vi "DAQ Loop.vi"(8 "error in":errorcluster, 10 "Queues":T1, 11 "Notifiers":T2) -> (0 "error out":errorcluster)   [LabVIEW 2014, in "DAQ.lvlib"]
uses:
  DAQ.lvlib
  support/Message Queue/Message Queue.lvlib
  TypeDefs/DAQ data.ctl
  <vilib>/ErrorRing/Error Ring.xnode
  PLC/PLC.lvlib
  <vilib>/Utility/error.llb/Error Cluster From Error Code.vi
  Support/Global names.vi
  Support/Message Queue/Message Cluster.ctl
  Support/Notifiers/Notifiers.ctl
  Support/Notifiers/Notifiers.lvlib
  Support/Message Queue/All Message Queues.ctl
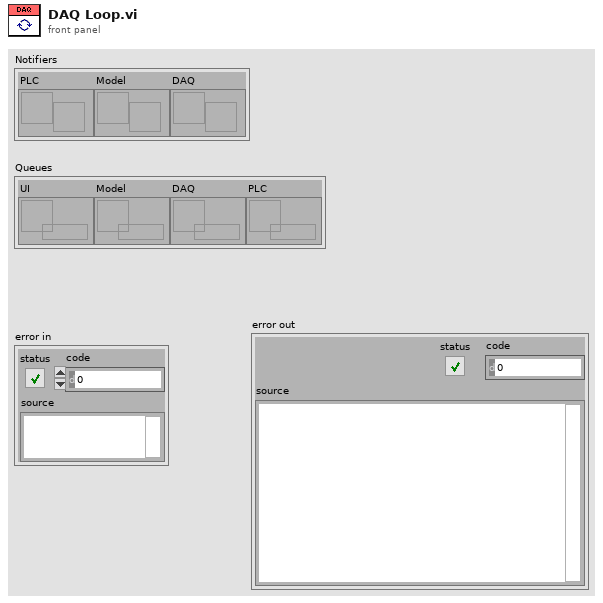
[diagram p1: front panel]
types:
  T1 = typedef "Message Queue.lvlib/All Message Queues.ctl" = cluster{"UI":refnum<queue>, "Model":refnum<queue>, "DAQ":refnum<queue>, "PLC":refnum<queue>}
  T2 = typedef "Notifiers.lvlib/Notifiers.ctl" = cluster{"PLC":refnum<notifier>, "Model":refnum<notifier>, "DAQ":refnum<notifier>}
  T3 = typedef "DAQ.lvlib/DAQ data.ctl" = cluster{"Power switch (DI)":cluster{"Channel":tag, "Data":bool}, "Dispose barrel (DI)":cluster{"Channel":tag, "Data":bool}, "Pump status (DO)":cluster{"Channel":tag, "Data":bool}, "Barrel position (AI)":cluster{"Channel":tag, "Data":dbl}}
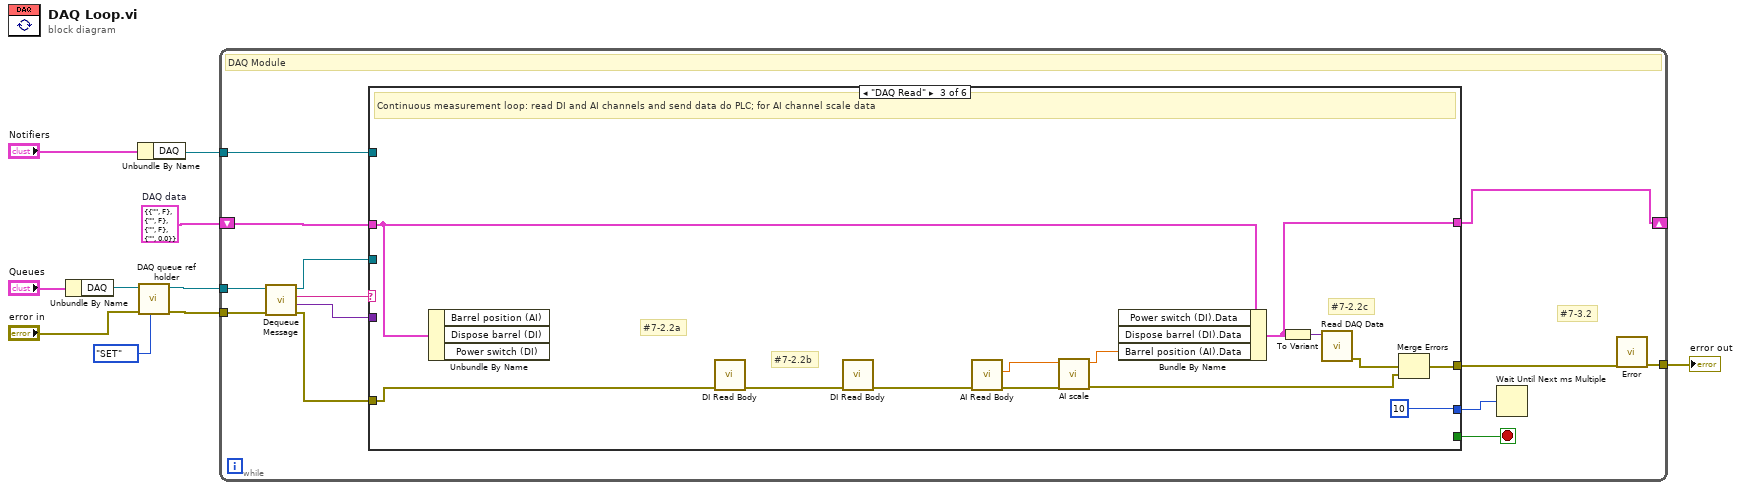
[diagram p0: block diagram]
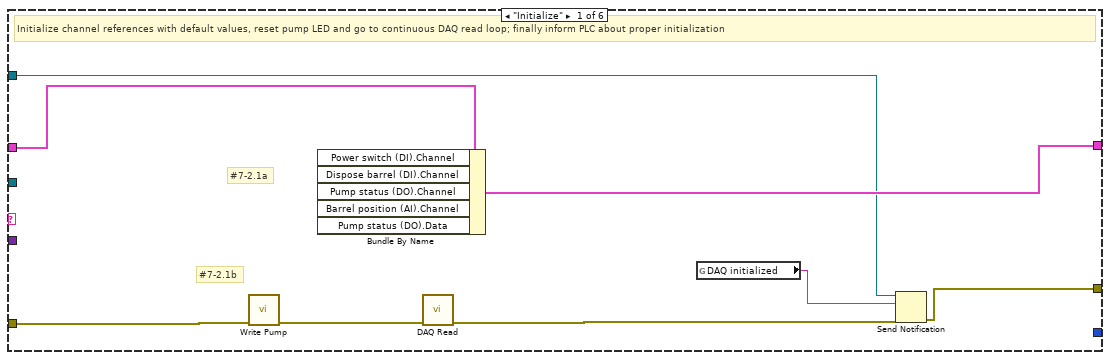
[diagram p2: hidden frame]
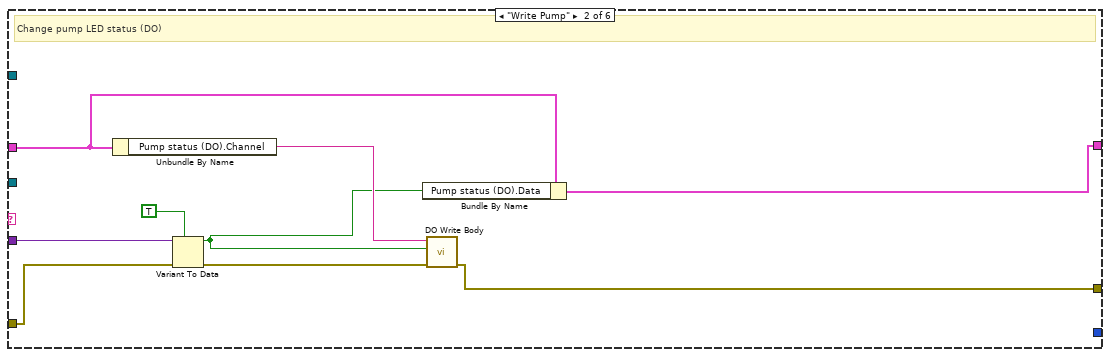
[diagram p3: hidden frame]
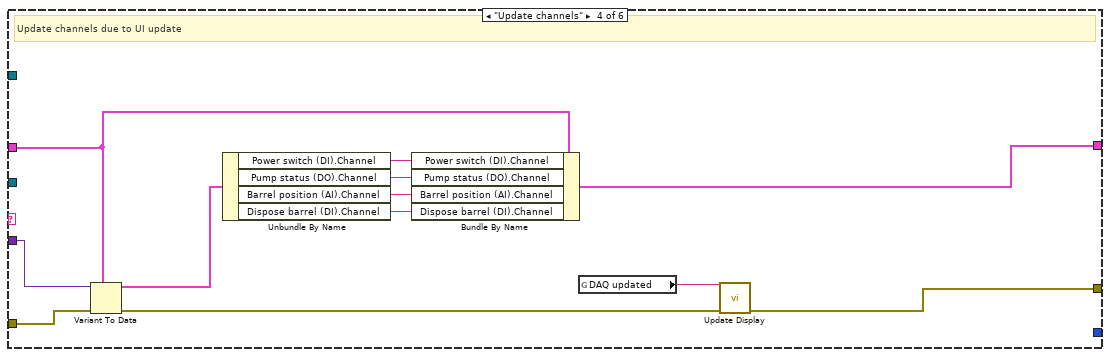
[diagram p4: hidden frame]
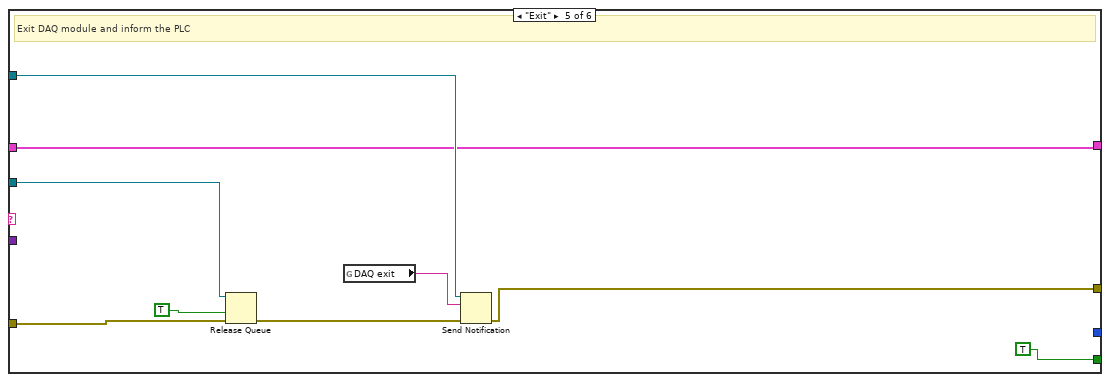
[diagram p5: hidden frame]
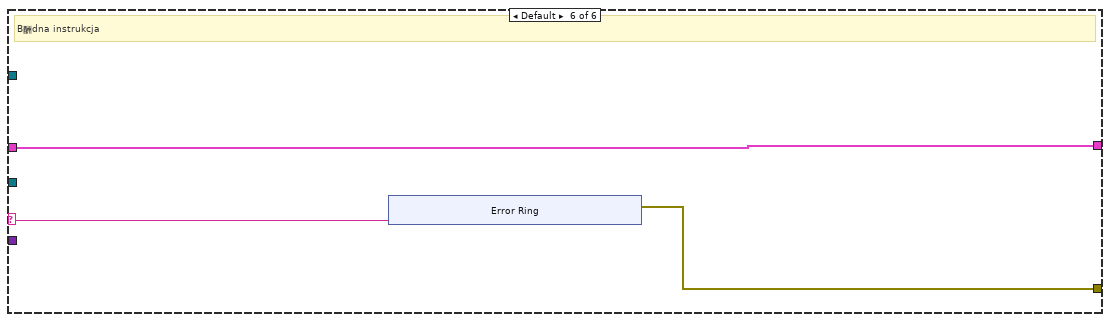
[diagram p6: hidden frame]
diagram:
  w10 = T3 {"Power switch (DI)"={"Channel"="", "Data"=FALSE}, "Dispose barrel (DI)"={"Channel"="", "Data"=FALSE}, "Pump status (DO)"={"Channel"="", "Data"=FALSE}, "Barrel position (AI)"={"Channel"="", "Data"=0.0}}  # DAQ data
  n1 = Unbundle By Name("Queues") -> ("DAQ"=w5:refnum<queue>)
  n2 = Unbundle By Name("Notifiers") -> ("DAQ"=w6:refnum<notifier>)
  n3 = call "DAQ queue ref holder.vi"("Action"=enum16{"GET", "SET"}."SET", "error in"="error in", "Message Queue In"=w5) -> ("error out"=w3:errorcluster, "Input Message Queue"=w4:refnum<queue>)  [unwired: 7 in]
  n4 = while {
    tunnel: w3 -> [w23]
    tunnel: w4 -> [w11]
    tunnel: w6 -> [w19]
    shift-right: [w18] -> _
    shift-left: w10 -> [w16]
    tunnel: [w14] -> w8
    stop <- w20 stop-if-true
    # "#7-3.2"
    # "DAQ Module"
    n5 = call "Dequeue Message.vi"("error in (no error)"=w23, "Message Queue"=w11) -> ("error out"=w22:errorcluster, "Message Data"=w21:variant, "Message"=w12:string, "dup Message Queue"=w13:refnum<queue>)  [unwired: 6 in]
    n6 = case shown="\"DAQ Read\"" w12 {
      selector: w12 -> [_ _ _ _ _ w76]
      tunnel: w22 -> [w28 w40 w46 w64 w68 _]
      tunnel: [w31 w32 w44 w56 w67 w75] -> w15
      tunnel: w21 -> [_ w39 _ w65 _ _]
      tunnel: [_ _ _ _ TRUE _] -> w20
      tunnel: w13 -> [_ _ _ _ w74 _]
      tunnel: w19 -> [w26 _ _ _ w73 _]
      tunnel: w16 -> [w30 w36 w51 w63 w69 w77]
      tunnel: [w29 w38 w48 w58 w69 w77] -> w18
      tunnel: [_ _ u32 10 ("millisecond multiple") _ _ _] -> w17
      frame "Initialize" {
        # "#7-2.1b"
        # "#7-2.1a"
        # "Initialize channel references with default values, reset pump LED and go to continuous DAQ read loop; finally inform PLC about proper initialization"
        n7 = call "Write Pump.vi"("error in"=w28) -> ("error out"=w27:errorcluster)  [unwired: 10 in]
        n8 = Bundle By Name(cluster=w30) -> (w29:T3)  [unwired: 5 in]
        n9 = call "DAQ Read.vi"("error in"=w27) -> ("error out"=w25:errorcluster)  [unwired: 10 in]
        n10 = global read "Global names.vi" "DAQ initialized"() -> (w24:string)
        n11 = Send Notification(notification=w24, notifier=w26, error in (no error)=w25) -> (error out=w31:errorcluster)  [unwired: 1 out]
      }
      frame "Write Pump" {
        # "Change pump LED status (DO)"
        n12 = Unbundle By Name(w36) -> ("Pump status (DO).Channel"=w37:tag)
        n13 = Variant To Data(error in=w40, type=TRUE, Variant=w39) -> (data=w34:bool, error out=w33:errorcluster)
        n14 = Bundle By Name(cluster=w36, "Pump status (DO).Data"=w34) -> (w38:T3)
        n15 = call "DO Write Body.vi"("error in"=w33, "data"=w34, "Channel"=w37) -> ("error out"=w32:errorcluster)  [unwired: 6 in]
      }
      frame "DAQ Read" {
        # "#7-2.2c"
        # "#7-2.2b"
        # "#7-2.2a"
        # "Continuous measurement loop: read DI and AI channels and send data do PLC; for AI channel scale data"
        n16 = Unbundle By Name(w51) -> ()  [unwired: 3 out]
        n17 = call "DI Read Body.vi"("error in"=w46) -> ("error out"=w53:errorcluster)  [unwired: 7 in, 1 out]
        n18 = call "DI Read Body.vi"("error in"=w53) -> ("error out"=w52:errorcluster)  [unwired: 7 in, 1 out]
        n19 = call "AI Read Body.vi"("error in"=w52) -> ("error out"=w45:errorcluster, "data"=w41:dbl)  [unwired: 7 in]
        n20 = call "AI scale.vi"("error in"=w45, "Data in"=w41) -> ("error out"=w42:errorcluster, "Data out"=w50:dbl)  [unwired: 8 in]
        n21 = Bundle By Name(cluster=w51, "Barrel position (AI).Data"=w50) -> (w48:T3)  [unwired: 2 in]
        n22 = To Variant(anything=w48) -> (Variant=w47:variant)
        n23 = call "Read DAQ Data.vi"("Message Data"=w47) -> ("error out"=w43:errorcluster)  [unwired: 10 in]
        n24 = Merge Errors(w43, w42) -> (w44:errorcluster)  [unwired: 1 in]
      }
      frame "Update channels" {
        # "Update channels due to UI update"
        n25 = Variant To Data(error in=w64, type=w63, Variant=w65) -> (data=w55:T3, error out=w57:errorcluster)
        n26 = Unbundle By Name(w55) -> ("Power switch (DI).Channel"=w62:tag, "Pump status (DO).Channel"=w61:tag, "Barrel position (AI).Channel"=w60:tag, "Dispose barrel (DI).Channel"=w59:tag)
        n27 = Bundle By Name(cluster=w63, "Power switch (DI).Channel"=w62, "Pump status (DO).Channel"=w61, "Barrel position (AI).Channel"=w60, "Dispose barrel (DI).Channel"=w59) -> (w58:T3)
        n28 = global read "Global names.vi" "DAQ updated"() -> (w54:string)
        n29 = call "Update Display.vi"("error in"=w57, "Message string"=w54) -> ("error out"=w56:errorcluster)  [unwired: 9 in]
      }
      frame "Exit" {
        # "Exit DAQ module and inform the PLC"
        n30 = Release Queue(queue=w74, force destroy? (F)=TRUE, error in (no error)=w68) -> (error out=w72:errorcluster)  [unwired: 2 out]
        n31 = global read "Global names.vi" "DAQ exit"() -> (w66:string)
        n32 = Send Notification(notification=w66, notifier=w73, error in (no error)=w72) -> (error out=w67:errorcluster)  [unwired: 1 out]
      }
      frame Default {
        # "B酬dna instrukcja"
        n33 = xnode "Error Ring"("parameter 0"=w76) -> ("error out"=w75:errorcluster)
      }
    }
    n34 = Wait Until Next ms Multiple(millisecond multiple=w17) -> ()  [unwired: 1 out]
    n35 = call "Error.vi"("error in"=w15) -> ("error out"=w14:errorcluster)  [unwired: 10 in]
  }
  "error out" <- w8
